vi "Write - All Errors Read.vi"(8 "Error In":errorcluster, 11 "All Errors Read?":bool) -> (0 "Error Out":errorcluster)   [LabVIEW 2023, in "Error Manager.lvlib"]
doc: "Blank VI with error handling."
uses:
  Error Manager.lvlib
  All Errors Read (library variable).vi
panel:
  # "Input\nInputs to the VI"
  # "Development\nControls or indicators that are useful for development or testing, but which are not outputs of the VI."
  # "Output\nOutputs of the VI"
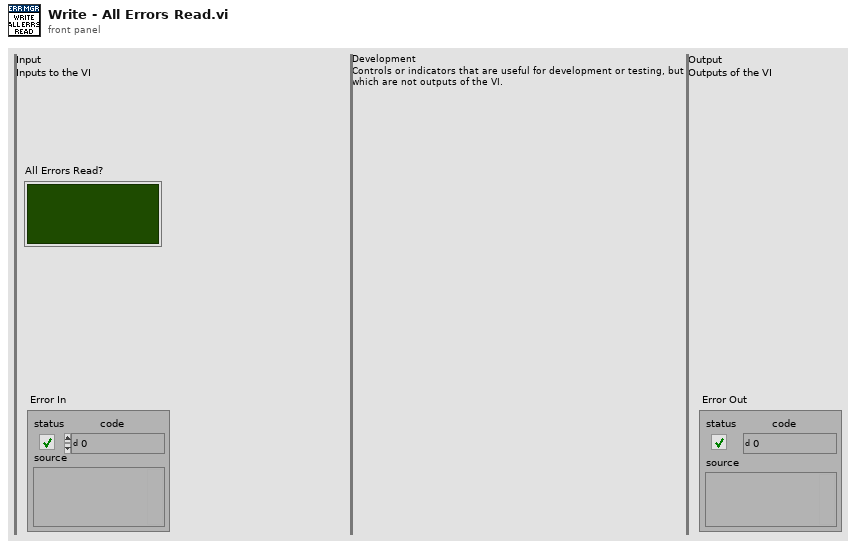
[diagram p1: front panel]
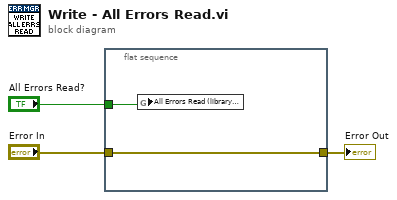
[diagram p0: block diagram]
diagram:
  n1 = flat-sequence {
    tunnel: [w5] -> w3
    tunnel: "Error In" -> [w5]
    tunnel: "All Errors Read?" -> [w4]
    frame #0 {
      n2 = global write "All Errors Read (library variable).vi" item#0(w4) -> ()
    }
  }
  "Error Out" <- w3
